vi "VsEP I-O Cal Config.vi"(0 "Stimulus":T5={"Rep rate (Hz)"=1.0, "Start (dB atten)"=20.0, "Stop (dB atten)"=0.0, "Step (dB)"=80.0}, 5 "Response":T2={"Accelerometer Sensitivity (mV/g)"=10000.0, "#Averages"=1024, "Time Window (ms)"=8.5, "Gain"=10000.0} {"Accelerometer Sensitivity (mV/g)" format="%_6g"}, 7 "Hidden":T4) -> (3 "Runtime":T3, 4 "RESPONSE":T1={"Grass Gain"=1, "#AVERAGES"=250, "Time Window (ms)"=25.0, "Fast Steps Threshold"=10000} {"Time Window (ms)" format="%.2f"}, 13 "Num Atten":i32, 14 "AI Sampling Interval (us)":dbl, 15 "error out":errorcluster)   [LabVIEW 2020]
uses:
  Typedefs/VsEPCal- Stimulus.ctl
  Typedefs/VsEP-Hidden Params.ctl
  epl-vi-lib/Signal Synthesis VIs/Controls/Gate XCtl/Gate Control.xctl
  Typedefs/VsEP-Runtime Data.ctl
  Typedefs/VsEPCal-Response.ctl
  Typedefs/VsEP-Response Control.ctl
  epl-vi-lib/Connection VIs/Type Defs/Input sources.ctl
  epl-vi-lib/Connection VIs/Type Defs/Output sources.ctl
  epl-vi-lib/Utility VIs/Math VIs/dB to Linear (scalar).vi
  epl-vi-lib/PXI DAQ VIs/DAQ Engine VIs/PXI Globals.vi
panel:
  in  "error in (no error)":errorcluster
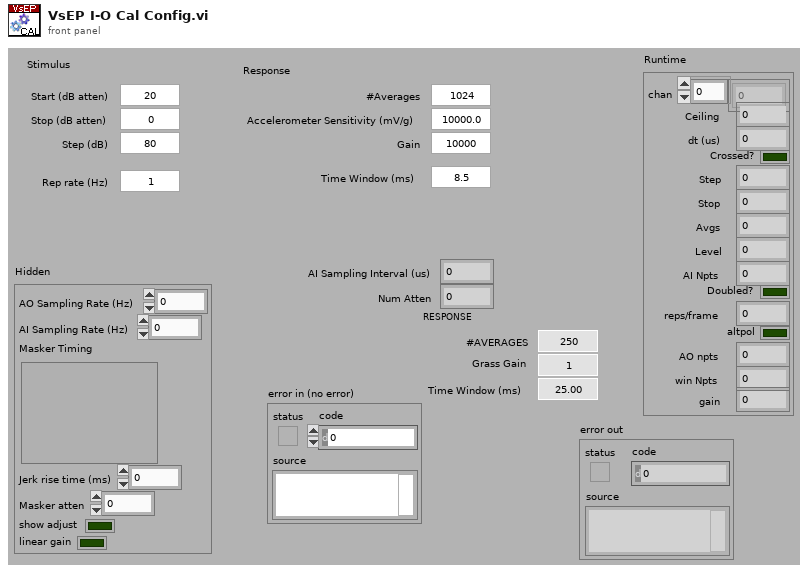
[diagram p1: front panel]
types:
  T1 = typedef "VsEP-Response Control.ctl" = cluster{"Grass Gain":i32, "#AVERAGES":i32, "Time Window (ms)":sgl, "Fast Steps Threshold":i32}
  T2 = typedef "VsEPCal-Response.ctl" = cluster{"Accelerometer Sensitivity (mV/g)":dbl, "#Averages":i32, "Time Window (ms)":dbl, "Gain":dbl}
  T3 = typedef "VsEP-Runtime Data.ctl" = cluster{"chan":i32[], "Ceiling":dbl, "dt (us)":dbl, "Crossed?":bool, "Step":dbl, "Stop":i32, "Avgs":i32, "Level":dbl, "AI Npts":i32, "Doubled?":bool, "reps/frame":i32, "altpol":bool, "AO npts":i32, "win Npts":i32, "gain":dbl}
  T4 = typedef "VsEP-Hidden Params.ctl" = cluster{"AO Sampling Rate (Hz)":dbl, "AI Sampling Rate (Hz)":dbl, "Masker Timing":cluster{"Active":bool, "Delay (ms)":dbl, "Width (ms)":dbl, "Ramp (ms)":dbl}, "Jerk rise time (ms)":dbl, "Masker atten":dbl, "show adjust":bool, "linear gain":bool}
  T5 = typedef "VsEPCal- Stimulus.ctl" = cluster{"Rep rate (Hz)":dbl, "Start (dB atten)":dbl, "Stop (dB atten)":dbl, "Step (dB)":dbl}
  T6 = typedef "Output sources.ctl" = u16
  T7 = typedef "Input sources.ctl" = u16
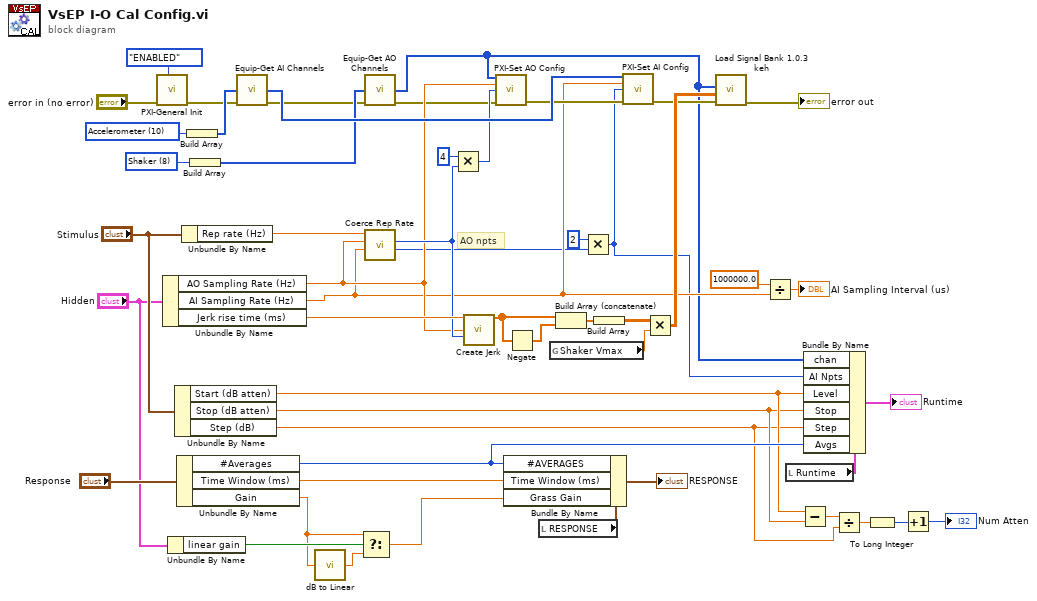
[diagram p0: block diagram]
diagram:
  w42 = T6 8 items=["--unused--", "Right primary", "Right secondary", "Left primary", "Left secondary", "Shocks", "Startle", "Background", "Shaker"] ("Ring")
  w47 = T7 10 items=["--unused--", "Probe Mic Right", "Probe Mic Left", "Cal Mic", "ABR", "CAP Right", "CAP Left", "Startle piezo", "Temperature", "Heart rate", "Accelerometer"] ("Ring")
  # "AO npts"
  n1 = call "PXI-General Init.vi"("Double Buffer Mode"=enum32{"OFF", "ENABLED", "FORCED"}."ENABLED", "error in (no error)"="error in (no error)") -> ("error out"=w45:errorcluster)  [unwired: 9 in]
  n2 = Unbundle By Name("Hidden") -> ("AO Sampling Rate (Hz)"=w32:dbl, "AI Sampling Rate (Hz)"=w22:dbl, "Jerk rise time (ms)"=w39:dbl)
  n3 = Unbundle By Name("Hidden") -> ("linear gain"=w4:bool)
  n4 = Unbundle By Name("Stimulus") -> ("Start (dB atten)"=w13:dbl, "Stop (dB atten)"=w12:dbl, "Step (dB)"=w10:dbl)
  n5 = Unbundle By Name("Response") -> ("#Averages"=w16:i32, "Time Window (ms)"=w14:dbl, "Gain"=w2:dbl)
  n6 = Unbundle By Name("Stimulus") -> ("Rep rate (Hz)"=w44:dbl)
  n7 = Build Array(w47) -> (w46:T7[])
  n8 = Build Array(w42) -> (w43:T6[])
  n9 = call "Equip-Get AI Channels.vi"("Inputs"=w46, "error in (no error)"=w45) -> ("AI Channels"=w52:i32[], "error out"=w28:errorcluster)  [unwired: 12 in]
  n10 = call-poly "dB to Linear.vi"("dB"=w2) -> ("linear"=w1:dbl)
  n11 = Select(t=w2, s=w4, f=w1) -> (s? t:f=w3:dbl)
  n12 = call "Equip-Get AO Channels.vi"("Outputs"=w43, "error in (no error)"=w28) -> ("AO Channels"=w6:i32[], "error out"=w30:errorcluster)  [unwired: 12 in]
  n13 = call "Coerce Rep Rate.vi"("AI sampling rate (Hz)"=w22, "AO sampling rate (Hz)"=w32, "Rep rate (Hz)"=w44) -> ("AI npts"=w21:i32, "AO npts"=w38:i32)  [unwired: 5 in, 2 out]
  n14 = Multiply(x=4, y=w38) -> (x*y=w33:i32)
  n15 = call "Create Jerk.vi"("Rise time (ms)"=w39, "Sampling Rate (Hz)"=w32, "Npts"=w38) -> ("Waveform"=w37:dbl[])  [unwired: 11 in, 1 out]
  n16 = call "PXI-Set AO Config.vi"("AO Channels"=w6, "Sampling Rate (Hz)"=w32, "Buffer Size"=w33, "error in (no error)"=w30) -> ("error out"=w31:errorcluster)  [unwired: 11 in]
  n17 = Negate(x=w37) -> (-x=w19:dbl[])
  n18 = local read "RESPONSE"() -> (w18:T1)
  n19 = Bundle By Name(cluster=w18, "#AVERAGES"=w16, "Time Window (ms)"=w14, "Grass Gain"=w3) -> (→"RESPONSE":T1)
  n20 = global read "PXI Globals.vi" "Shaker Vmax"() -> (w36:dbl)
  n21 = Build Array (concatenate)(w37, w19) -> (w35:dbl[])
  n22 = Multiply(x=2, y=w21) -> (x*y=w20:i32)
  n23 = Build Array(w35) -> (w27:dbl[][])
  n24 = call "PXI-Set AI Config.vi"("AI Channels"=w52, "Sampling Rate (Hz)"=w22, "Buffer Size"=w20, "error in (no error)"=w31) -> ("error out"=w29:errorcluster)  [unwired: 11 in]
  n25 = Multiply(x=w27, y=w36) -> (x*y=w34:dbl[][])
  n26 = call "Load Signal Bank 1.0.3 keh.vi"("error in (no error)"=w29, "Input array"=w34, "Active AO Array"=w6) -> ("error out"=→"error out":errorcluster)  [unwired: 6 in, 2 out]
  n27 = Divide(x=1000000.0, y=w22) -> (x/y=→"AI Sampling Interval (us)":dbl)
  n28 = local read "Runtime"() -> (w25:T3)
  n29 = Subtract(x=w13, y=w12) -> (x-y=w11:dbl)
  n30 = Bundle By Name(cluster=w25, "chan"=w6, "AI Npts"=w20, "Level"=w13, "Stop"=w12, "Step"=w10, "Avgs"=w16) -> (→"Runtime":T3)
  n31 = Divide(x=w11, y=w10) -> (x/y=w9:dbl)
  n32 = To Long Integer(number=w9) -> (32bit integer=w8:i32)
  n33 = Increment(x=w8) -> (x+1=→"Num Atten":i32)
